vi "Create.vi"(9 "Actor":refnum<class "Actor.lvclass">, 10 "Alias":string, 11 "Create in":refnum<class "Create.lvclass">) -> (3 "Create out":refnum<class "Create.lvclass">)   [LabVIEW 2021, in "Create.lvlib" / "Create.lvclass"]
uses:
  Create.lvclass
  Actor/Actor.lvclass
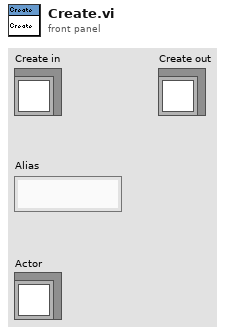
[diagram p1: front panel]
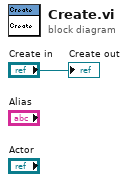
[diagram p0: block diagram]
diagram:
  "Create out" <- "Create in"
